vi "circuitosecuencial.vi"() -> ()   [LabVIEW 2018]
panel:
  in  "stop":bool
  in  "Slide":dbl(slide) scale=1.0..1000.0
  in  "SENTIDO":bool
  out "?":bool
  out "?":bool
  out "?":bool
  out "?":bool
  # "SECUENCIA"
  # "DAVID FLORES"
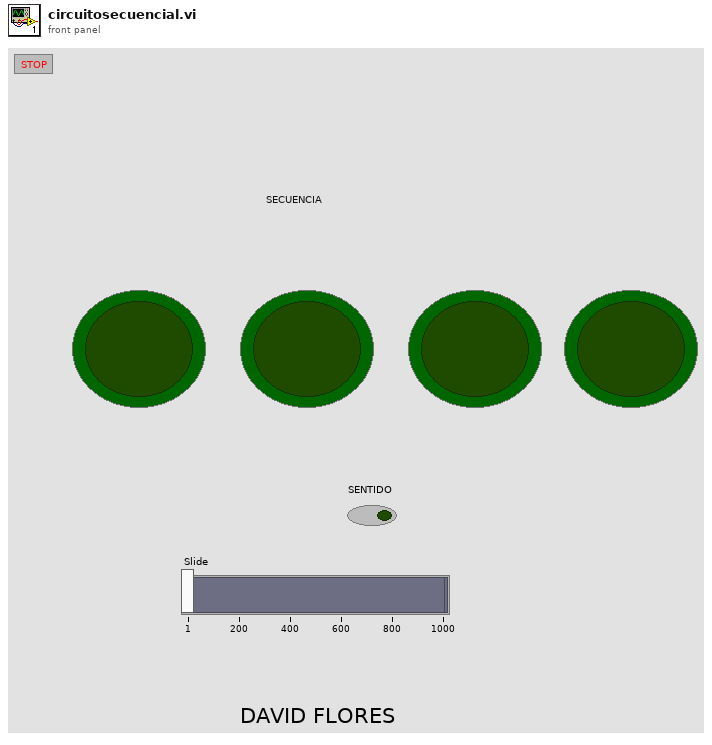
[diagram p1: front panel]
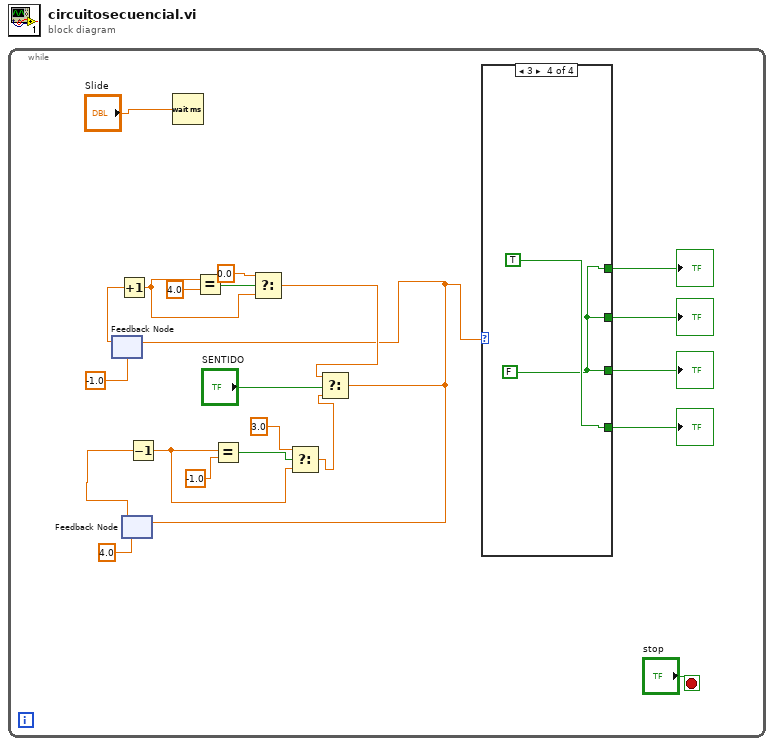
[diagram p0: block diagram]
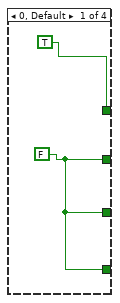
[diagram p2: hidden frame]
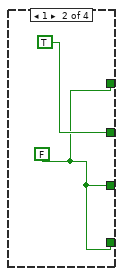
[diagram p3: hidden frame]
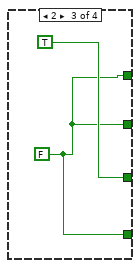
[diagram p4: hidden frame]
diagram:
  n1 = while {
    stop <- "stop" stop-if-true
    n2 = feedback #1(-1.0) -> (w21:dbl)
    n3 = Increment(x=w21) -> (x+1=w16:dbl)
    n4 = feedback #2(4.0) -> (w14:dbl)
    n5 = Decrement(x=w14) -> (x-1=w9:dbl)
    n6 = Wait (ms)(milliseconds to wait="Slide") -> ()  [unwired: 1 out]
    n7 = Equal?(x=w16, y=4.0) -> (x = y?=w18:bool)
    n8 = Equal?(x=w9, y=-1.0) -> (x = y?=w11:bool)
    n9 = Select(t=0.0, s=w18, f=w16) -> (s? t:f=w7:dbl)
    n10 = Select(t=3.0, s=w11, f=w9) -> (s? t:f=w6:dbl)
    n11 = Select(t=w7, s="SENTIDO", f=w6) -> (s? t:f=w5:dbl)
    n12 = feedback-in #1(w5) -> ()
    n13 = feedback-in #2(w5) -> ()
    n14 = case shown="3" w5 {
      tunnel: [TRUE w25 w27 w29] -> w4
      tunnel: [w23 TRUE w27 w29] -> w3
      tunnel: [w23 w25 w27 TRUE] -> w2
      tunnel: [w23 w25 TRUE w29] -> w1
      frame 0, Default {
        w23 = FALSE
      }
      frame 1 {
        w25 = FALSE
      }
      frame 2 {
        w27 = FALSE
      }
      frame 3 {
        w29 = FALSE
      }
    }
    "?" <- w4
    "?" <- w3
    "?" <- w1
    "?" <- w2
  }
